vi "Test.vi"() -> ()   [LabVIEW 2015, in "Touch_keyboard.lvlib"]
uses:
  Touch_keyboard.lvlib
panel:
  in  "Keyboard":bool
  in  "stop":bool
  in  "Numeric":dbl
  in  "String":string
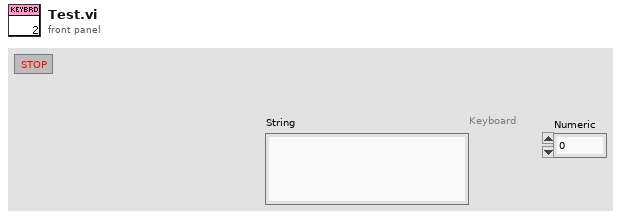
[diagram p1: front panel]
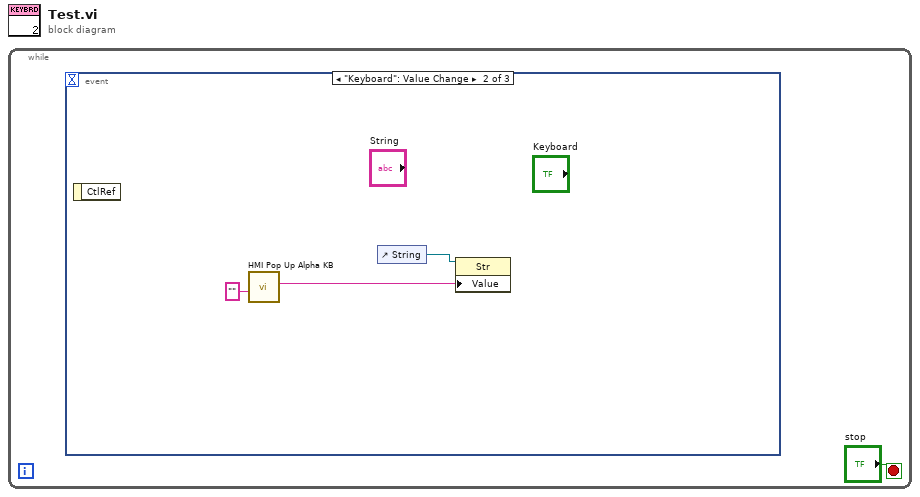
[diagram p0: block diagram]
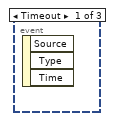
[diagram p2: hidden frame]
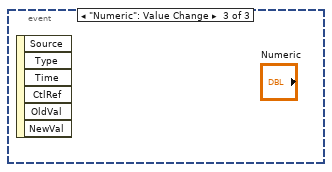
[diagram p3: hidden frame]
diagram:
  n1 = while {
    stop <- "stop" stop-if-true
    n2 = event shown="[1] \"Keyboard\": Value Change" {
      selector: _ -> [_ _ _]
      dyn-events: _ -> [_ _ _]
      timeout: _ -> [_ _ _]
      event Timeout {
        n3 = event-data() -> ()  [unwired: 1 in, 3 out]
      }
      event "Keyboard": Value Change {
        n4 = event-data() -> ()  [unwired: 1 in, 1 out]
        n5 = call "HMI Pop Up Alpha KB.vi"("Text"="") -> ("String Out"=w4:string)  [unwired: 8 in, 2 out]
        n6 = control-ref of="String"() -> (w3:refnum<vi>)
        n7 = property class="Str"(reference=w3, "Value"=w4) -> ()  [unwired: 1 in, 2 out]
      }
      event "Numeric": Value Change {
        n8 = event-data() -> ()  [unwired: 1 in, 6 out]
      }
    }
  }
